vi "setSerializedData.vi"(0 "reference":refnum<class "SystemNode.lvclass">, 1 "parent":refnum<class "AbstractNode.lvclass">, 2 "children":refnum<class "AbstractNode.lvclass">[](array[class]), 3 "xmlOut":string, 5 "error in (no error)":errorcluster) -> (14 "reference out":refnum<class "SystemNode.lvclass">, 19 "error out":errorcluster)   [LabVIEW 2014, in "SystemNode.lvclass"]
doc: "setSerializedData"
uses:
  <resource>/Framework/Providers/Open_GDS/UML/SystemNode_class/SystemNode.lvclass
  <resource>/Framework/Providers/Open_GDS/UML/AbstractNode_class/AbstractNode.lvclass
  <resource>/Framework/Providers/Open_GDS/UML/General/Rectangle/Rectangle Rectangle2D.ctl
  <resource>/Framework/Providers/Open_GDS/UML/MultiLineString_class/MultiLineString.lvclass
  <resource>/Framework/Providers/Open_GDS/UML/RectangularNode_class/RectangularNode.lvclass
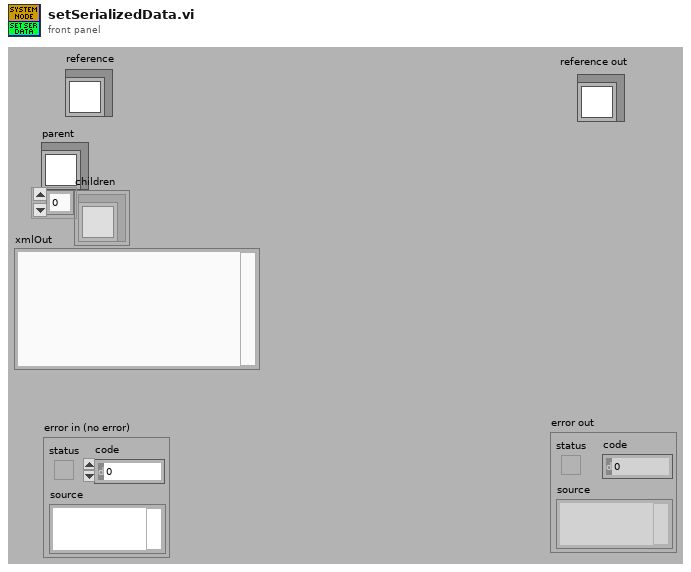
[diagram p1: front panel]
types:
  T1 = typedef "Rectangle Rectangle2D.ctl" = cluster{"x":dbl, "y":dbl, "width":dbl, "height":dbl}
  T2 = cluster{"Base class":cluster{"Base class":cluster{"parent":refnum<k1>, "children":refnum<k1>[]}, "bounds":T1}, "contents":refnum<k1>, "DEFAULT_WIDTH":i32, "DEFAULT_HEIGHT":i32, "NAME_GAP":i32, "XGAP":i32, "YGAP":i32}
  T3 = cluster{"Attributes":cluster{"Base class":cluster{"Base class":cluster{"parent":refnum<k1>, "children":refnum<k1>[]}, "bounds":T1}, "contents":refnum<k1>, "DEFAULT_WIDTH":i32, "DEFAULT_HEIGHT":i32, "NAME_GAP":i32, "XGAP":i32, "YGAP":i32}, string}
  T4 = typedef "SystemNode.lvclass/ObjectAttributes.ctl" = cluster{"contents":refnum<class "MultiLineString.lvclass">, "DEFAULT_WIDTH":i32, "DEFAULT_HEIGHT":i32, "NAME_GAP":i32, "XGAP":i32, "YGAP":i32}
  T5 = typedef "RectangularNode.lvclass/ObjectAttributes.ctl" = cluster{"bounds":T1}
  T6 = typedef "AbstractNode.lvclass/ObjectAttributes.ctl" = cluster{"parent":refnum<class "AbstractNode.lvclass">, "children":refnum<class "AbstractNode.lvclass">[], "Hidden":bool}
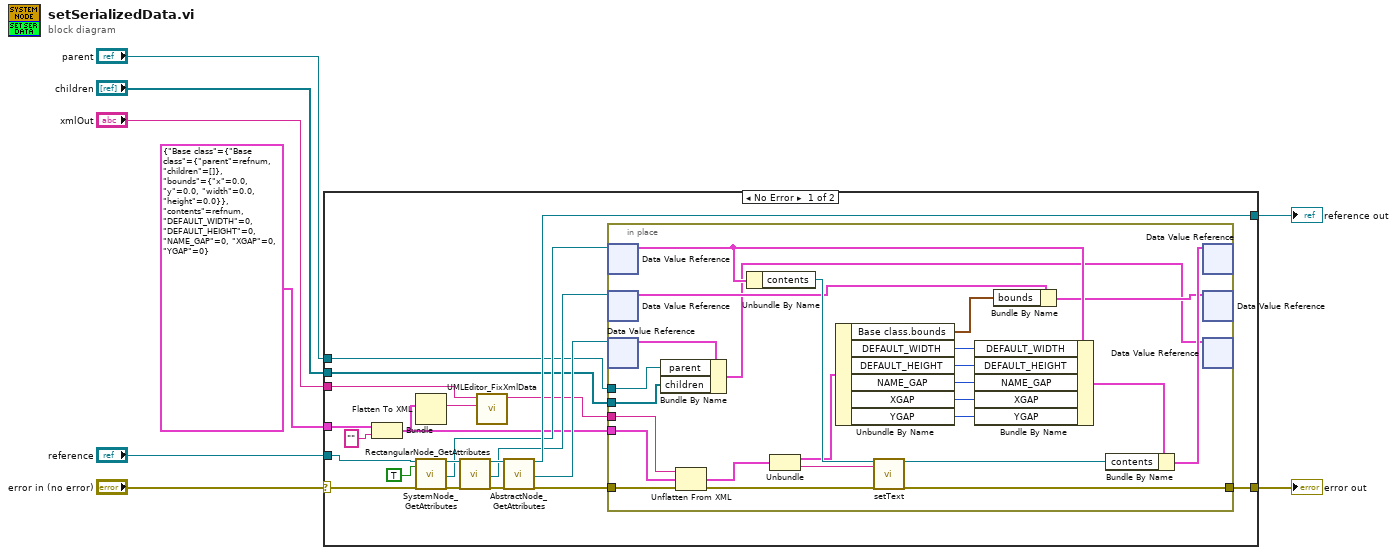
[diagram p0: block diagram]
diagram:
  n1 = case shown="No Error" "error in (no error)" {
    selector: "error in (no error)" -> [w28 w55]
    tunnel: "reference" -> [w29 w56]
    tunnel: [w27 w55] -> w6
    tunnel: [w26 w56] -> w5
    tunnel: "xmlOut" -> [w10 _]
    tunnel: "parent" -> [w12 _]
    tunnel: "children" -> [w11 _]
    tunnel: T2 {"Base class"={"Base class"={"parent"=refnum, "children"=[]}, "bounds"={"x"=0.0, "y"=0.0, "width"=0.0, "height"=0.0}}, "contents"=refnum, "DEFAULT_WIDTH"=0, "DEFAULT_HEIGHT"=0, "NAME_GAP"=0, "XGAP"=0, "YGAP"=0} ("Attributes") -> [w24 _]
    frame No Error {
      n2 = Bundle("Attributes"=w24, "") -> (w13:T3)  [unwired: 1 out]
      n3 = Flatten To XML(anything=w13) -> (xml string=w23:string)
      n4 = call <resource>:"SystemNode_GetAttributes.vi"("reference in"=w29, "OnlyGetDvrReference(False)"=TRUE, "error in (no error)"=w28) -> ("reference out"=w21:refnum<class "SystemNode.lvclass">, "DataRef"=w17:refnum<data-value>, "error out"=w20:errorcluster)  [unwired: 13 in, 1 out]
      n5 = call <resource>:"RectangularNode_GetAttributes.vi"("reference in"=w21, "error in (no error)"=w20) -> ("reference out"=w19:refnum<class "SystemNode.lvclass">, "DataRef"=w16:refnum<data-value>, "error out"=w18:errorcluster)  [unwired: 14 in, 1 out]
      n6 = call <resource>:"UMLEditor_FixXmlData.vi"("XmlTemplateIn"=w23, "xmlIn"=w10) -> ("XML OUt"=w9:string)  [unwired: 9 in]
      n7 = call <resource>:"AbstractNode_GetAttributes.vi"("reference in"=w19, "error in (no error)"=w18) -> ("reference out"=w26:refnum<class "SystemNode.lvclass">, "DataRef"=w15:refnum<data-value>, "error out"=w14:errorcluster)  [unwired: 14 in, 1 out]
      n8 = in-place {
        in-place-border: [w40] -> w27
        in-place-border: w14 -> [w37]
        in-place-border: w13 -> [w36]
        in-place-border: w9 -> [w35]
        in-place-border: w12 -> [w32]
        in-place-border: w11 -> [w31]
        n9 = in-place-dvr #1(w17) -> (w54:T4)  [unwired: 1 out]
        n10 = in-place-dvr #2(w16) -> (w38:T5)  [unwired: 1 out]
        n11 = in-place-dvr #3(w15) -> (w33:T6)  [unwired: 1 out]
        n12 = Bundle By Name(cluster=w33, "parent"=w32, "children"=w31) -> (w30:T6)
        n13 = Unflatten From XML(xml string=w35, type=w36, error in (no error)=w37) -> (value=w39:T3, error out=w41:errorcluster)
        n14 = Unbundle By Name(w54) -> ("contents"=w47:refnum<class "MultiLineString.lvclass">)
        n15 = Unbundle(w39) -> ("Attributes"=w44:T2, w42:string)
        n16 = Unbundle By Name(w44) -> ("Base class.bounds"=w43:T1, "DEFAULT_WIDTH"=w53:i32, "DEFAULT_HEIGHT"=w52:i32, "NAME_GAP"=w51:i32, "XGAP"=w50:i32, "YGAP"=w49:i32)
        n17 = call-dynamic "setText.vi"("reference"=w47, "text"=w42, "error in (no error)"=w41) -> ("reference out"=w46:refnum<class "MultiLineString.lvclass">, "error out"=w40:errorcluster)  [unwired: 15 out]
        n18 = Bundle By Name(cluster=w54, "DEFAULT_WIDTH"=w53, "DEFAULT_HEIGHT"=w52, "NAME_GAP"=w51, "XGAP"=w50, "YGAP"=w49) -> (w48:T4)
        n19 = Bundle By Name(cluster=w38, "bounds"=w43) -> (w34:T5)
        n20 = Bundle By Name(cluster=w48, "contents"=w46) -> (w45:T4)
        n21 = in-place-dvr #1(w45) -> ()  [unwired: 2 out]
        n22 = in-place-dvr #2(w34) -> ()  [unwired: 2 out]
        n23 = in-place-dvr #3(w30) -> ()  [unwired: 2 out]
      }
    }
    frame Error {
    }
  }
  "reference out" <- w5
  "error out" <- w6
